vi "DestroySelfReference.vi"(8 "error in (no error)":errorcluster, 11 "OPA.OrpheusHP":refnum<class "OPA.OrpheusHP.lvclass">) -> (0 "error out":errorcluster, 3 "OPA.OrpheusHP out":refnum<class "OPA.OrpheusHP.lvclass">)   [LabVIEW 2017, in "OPA.OrpheusHP.lvclass"]
doc: "JKI State Machine Objects (SMO) 1.0.0.5\nJKI - JKI\nCopyright (c) 2016, JKI"
uses:
  OPA.OrpheusHP.lvclass
  OPA.OrpheusHP.lvclass/OPA.OrpheusHP.ctl
  OPA/OPA.lvclass
panel:
  # "For instructions on how to use the JKI State Machine Objects, examples and video tutorials, visit:\nhttp://jki.net/state-machine-objects/\n\nJKI State Machine Objects™\nhttp://jki.net/state-machine-objects/\nCopyright (C) 2005-2015, JKI <info@jki.net>\nALL RIGHTS RESERVED"
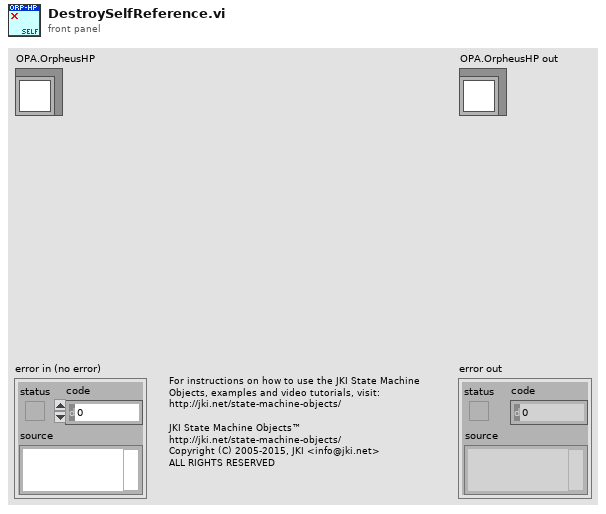
[diagram p1: front panel]
types:
  T1 = typedef "OPA.OrpheusHP.lvclass/PrivateData--Ref.ctl" = refnum<data-value>
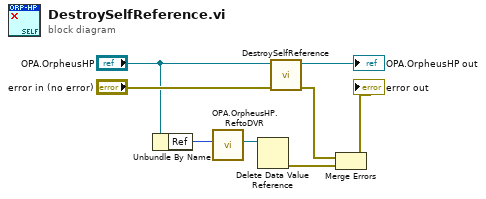
[diagram p0: block diagram]
diagram:
  n1 = Unbundle By Name("OPA.OrpheusHP") -> ("Ref"=w2:u32)
  n2 = call "OPA.OrpheusHP.ReftoDVR.vi"("Ref"=w2) -> ("Ref"=w1:T1)  [unwired: 10 in]
  n3 = Delete Data Value Reference(data value reference=w1) -> (error out=w5:errorcluster)  [unwired: 1 in, 1 out]
  n4 = call-parent "DestroySelfReference.vi"("error in (no error)"="error in (no error)", "OPA"="OPA.OrpheusHP") -> ("error out"=w4:errorcluster, "OPA out"=→"OPA.OrpheusHP out":refnum<class "OPA.OrpheusHP.lvclass">)  [unwired: 8 in]
  n5 = Merge Errors(w4, w5) -> (→"error out":errorcluster)
